vi "Handle Message.vi"(8 "error in (no error)":errorcluster, 9 "TcpPayload":T1, 11 "RemoteCommandable in":refnum<class "RemoteCommandable.lvclass">) -> (0 "error out":errorcluster, 3 "RemoteCommandable out":refnum<class "RemoteCommandable.lvclass">)   [LabVIEW 2020, in "Volatus.lvlib" / "RemoteCommandable.lvclass"]
uses:
  RemoteCommandable.lvclass
  lv-vecto/Vecto/proto/TcpPayload/Data.ctl
  lv-vecto/Vecto/proto/TcpPayload/TcpPayload.lvlib
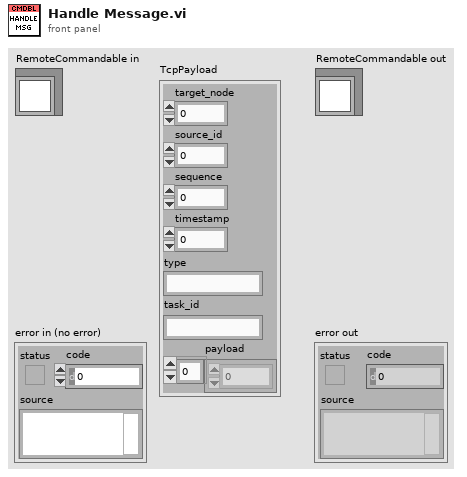
[diagram p1: front panel]
types:
  T1 = typedef "TcpPayload.lvlib/Data.ctl" = cluster{"target_node":u32, "source_id":u32, "sequence":u32, "timestamp":u64, "type":string, "task_id":string, "payload":u8[]}
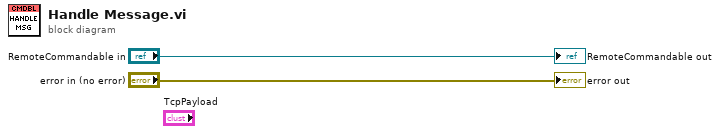
[diagram p0: block diagram]
diagram:
  "error out" <- "error in (no error)"
  "RemoteCommandable out" <- "RemoteCommandable in"
